vi "workingPicGlobal.vi"(5 "File Path":path, 6 "Enum":T2(ring)) -> (0 "error out":errorcluster, 1 "title":string, 2 "Image Out":T1)   [LabVIEW 2009]
uses:
  <vilib>/vision/Image Controls.llb/IMAQ Image.ctl
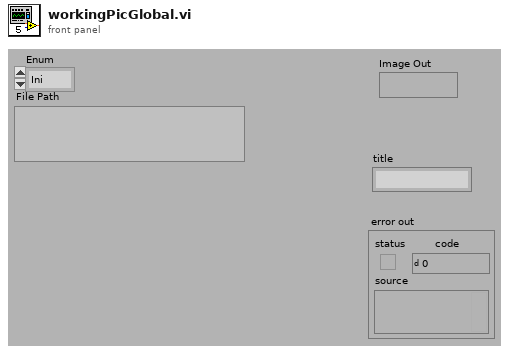
[diagram p1: front panel]
types:
  T1 = typedef "IMAQ Image.ctl" = refnum<image>
  T2 = enum16{"Ini", "Load", "Save as", "Get", "draw", "dump"}
  T3 = cluster{"Read Raw File":i32, "File Data Type":u32, "Offset to Data":i32, "Use Min Max":enum32{"Don't use min max", "Use file values", "Use optional values"}, "Optional Min Value":sgl, "Optional Max Value":sgl, "Byte Order":enum32{"Big endian (Motorola)", "Little endian (Intel)"}}
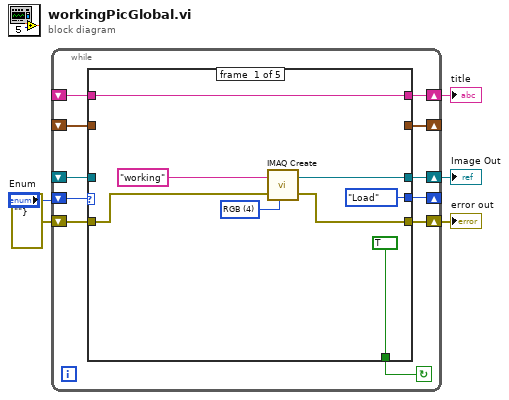
[diagram p0: block diagram]
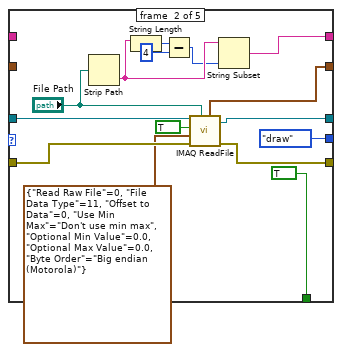
[diagram p2: hidden frame]
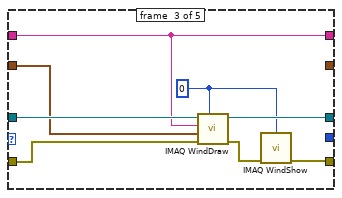
[diagram p3: hidden frame]
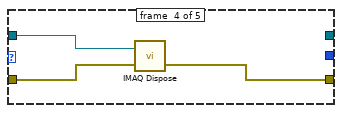
[diagram p4: hidden frame]
diagram:
  n1 = while {
    shift-right: [w16] -> w4
    shift-left: _ -> [w15]
    shift-right: [w13] -> _
    shift-left: "Enum" -> [w14]
    shift-right: [w11] -> _
    shift-left: _ -> [w10]
    shift-right: [w9] -> w1
    shift-left: errorcluster {"status"=FALSE, "code"=0, "source"=""} ("error out") -> [w8]
    shift-right: [w7] -> w3
    shift-left: _ -> [w6]
    stop <- w12 continue-if-true
    n2 = case shown="\"draw\"" w14 {
      tunnel: [w24 w36 w46 _ w52] -> w16
      tunnel: w15 -> [_ w39 w47 w48 w52]
      tunnel: [enum16{"Ini", "Load", "Save as", "Get", "draw"}."Load" ("Enum") enum16{"Ini", "Load", "Save as", "Get", "draw"}."draw" ("Enum") _ _ _] -> w13
      tunnel: [TRUE TRUE _ _ _] -> w12
      tunnel: [_ w28 _ _ w53] -> w11
      tunnel: w10 -> [_ _ w45 _ w53]
      tunnel: [w19 w34 w41 w49 w51] -> w9
      tunnel: w8 -> [w18 w35 w44 w50 w51]
      tunnel: [w17 w25 w43 _ w54] -> w7
      tunnel: w6 -> [w17 _ w43 _ w54]
      frame #0 {
        w22 = u32 4 items=["8 bits", "16 bits", "Float", "Complex", "RGB", "HSL"] ("Image Type")
        n3 = call "IMAQ Create"("Image Name"="working", "Image Type"=w22, "error in (no error)"=w18) -> ("New Image"=w24:T1, "error out"=w19:errorcluster)  [unwired: 2 in]
      }
      frame #1 {
        n4 = Strip Path(path="File Path") -> (name=w27:string)  [unwired: 1 out]
        n5 = String Length(string=w27) -> (length=w30:i32)
        n6 = Subtract(x=w30, y=4) -> (x-y=w26:i32)
        n7 = call "IMAQ ReadFile"("File Path"="File Path", "error in (no error)"=w35, "File Options"=T3 {"Read Raw File"=0, "File Data Type"=11, "Offset to Data"=0, "Use Min Max"=enum."Don't use min max", "Optional Min Value"=0.0, "Optional Max Value"=0.0, "Byte Order"=enum."Big endian (Motorola)"}, "Load Color Palette? (No)"=TRUE, "Image"=w39) -> ("error out"=w34:errorcluster, "Image Out"=w36:T1, "Color Palette out"=w28:cluster{"Red":u8, "Green":u8, "Blue":u8}[])  [unwired: 2 in, 2 out]
        n8 = String Subset(string=w27, length (rest)=w26) -> (substring=w25:string)  [unwired: 1 in]
      }
      frame #2 {
        w40 = 0 ("Window Number (0...15)")
        n9 = call "IMAQ WindDraw"("Window Number (0...15)"=w40, "error in (no error)"=w44, "Color Palette"=w45, "Title"=w43, "Image"=w47) -> ("error out"=w42:errorcluster, "Image Out (duplicate)"=w46:T1)  [unwired: 5 in]
        n10 = call "IMAQ WindShow"("error in (no error)"=w42, "Window Number (0...15)"=w40) -> ("error out"=w41:errorcluster)  [unwired: 4 in, 2 out]
      }
      frame #3 {
        n11 = call "IMAQ Dispose"("Image"=w48, "error in (no error)"=w50) -> ("error out"=w49:errorcluster)  [unwired: 4 in]
      }
      frame #4 {
      }
    }
  }
  "Image Out" <- w4
  "title" <- w3
  "error out" <- w1
